vi "Afficheur - Copie.vi"() -> ()   [LabVIEW 2013]
uses:
  <vilib>/DAQmx/read.llb/DAQmx Read (Analog Wfm 1Chan NSamp).vi
  <vilib>/DAQmx/create/channels.llb/DAQmx Create Channel (AI-Voltage-Basic).vi
  <vilib>/DAQmx/configure/timing.llb/DAQmx Timing (Sample Clock).vi
  <vilib>/measure/matone.llb/Extract Single Tone Information 1 Chan.vi
  <vilib>/DAQmx/miscellaneous.llb/DAQmx Fill In Error Info.vi
  <vilib>/express/express analysis/Spectral/Block/exnSpectralBlock spectral measurements PSD poly.vi
  <vilib>/express/express analysis/Spectral/Block/exnSpectralBlock spectral measurements PSD WFM.vi
  <vilib>/express/express analysis/Spectral/XNode/ExpressSpectralMeasurementsBlockNode.xnode
  <vilib>/measure/NI_MAPro.lvlib
panel:
  out "indice fractionnaire ou x":dbl
  out "Y":dbl[](array[numeric])
  out "taille(s) 2":i32
  out "taille(s)":i32
  out "x*y":dbl
  out "Final Waveform":waveform(dbl)(graph)
  in  "TA":dbl
  out "signal 2":dbl[](graph)
  out "Valeur efficace":dbl
  out "?":cluster{"f0":dbl, "df":dbl, "magnitude":dbl[]}(graph)
  out "mean":dbl caption="moyenne" format="%0.2f"
  out "signal":waveform(dbl)(graph)
  out "Fréquence":dbl
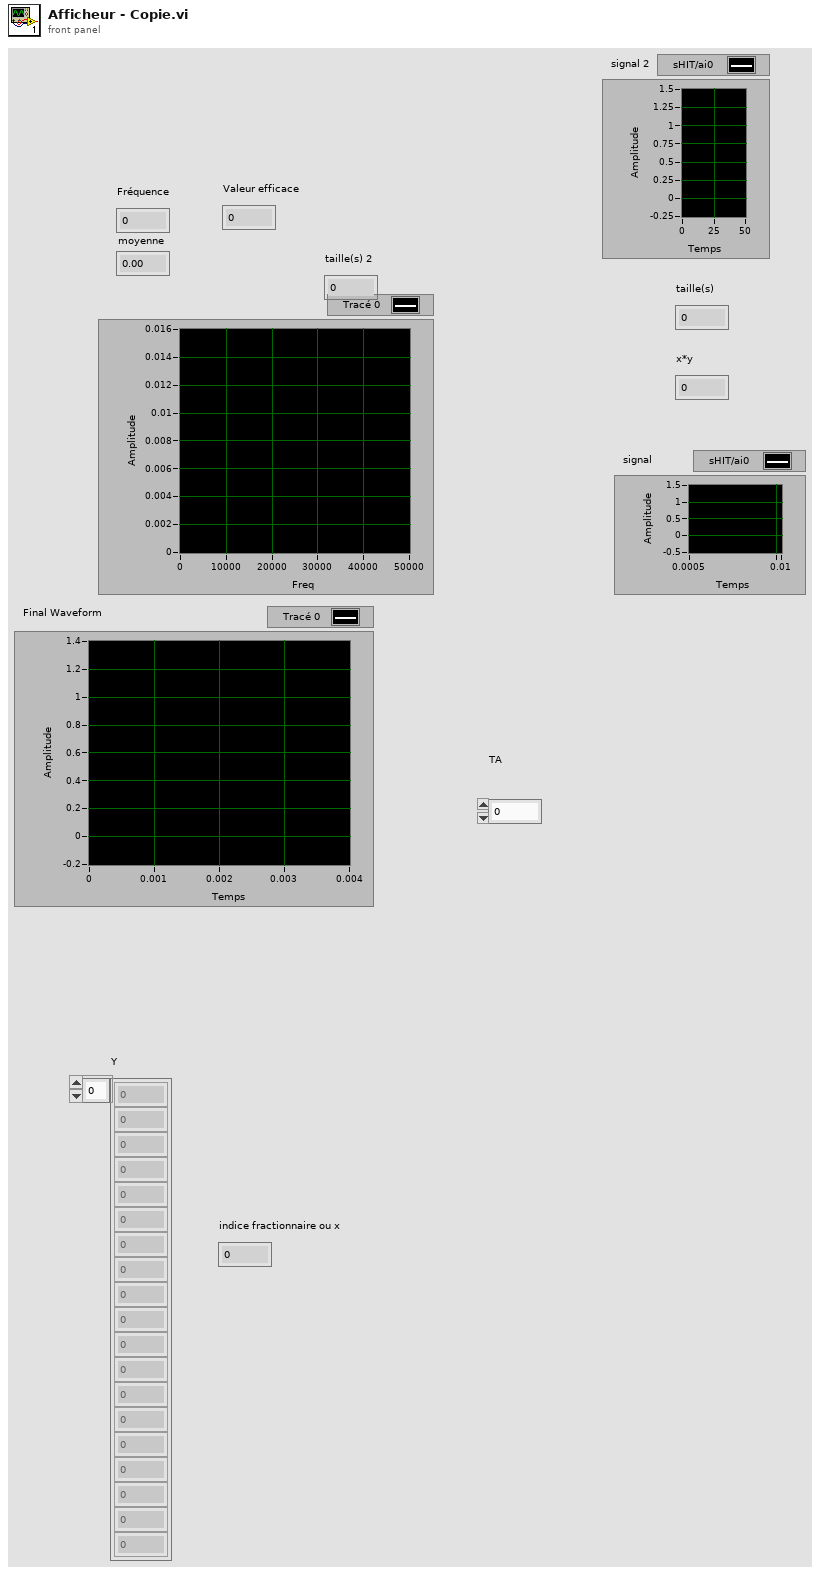
[diagram p1: front panel]
types:
  T1 = cluster{"averaging mode":u16, "weighting mode":u16, "number of averages":u32}
  T2 = cluster{"dB On (F)":bool, "unwrap phase (F)":bool, "convert to degree (F)":bool}
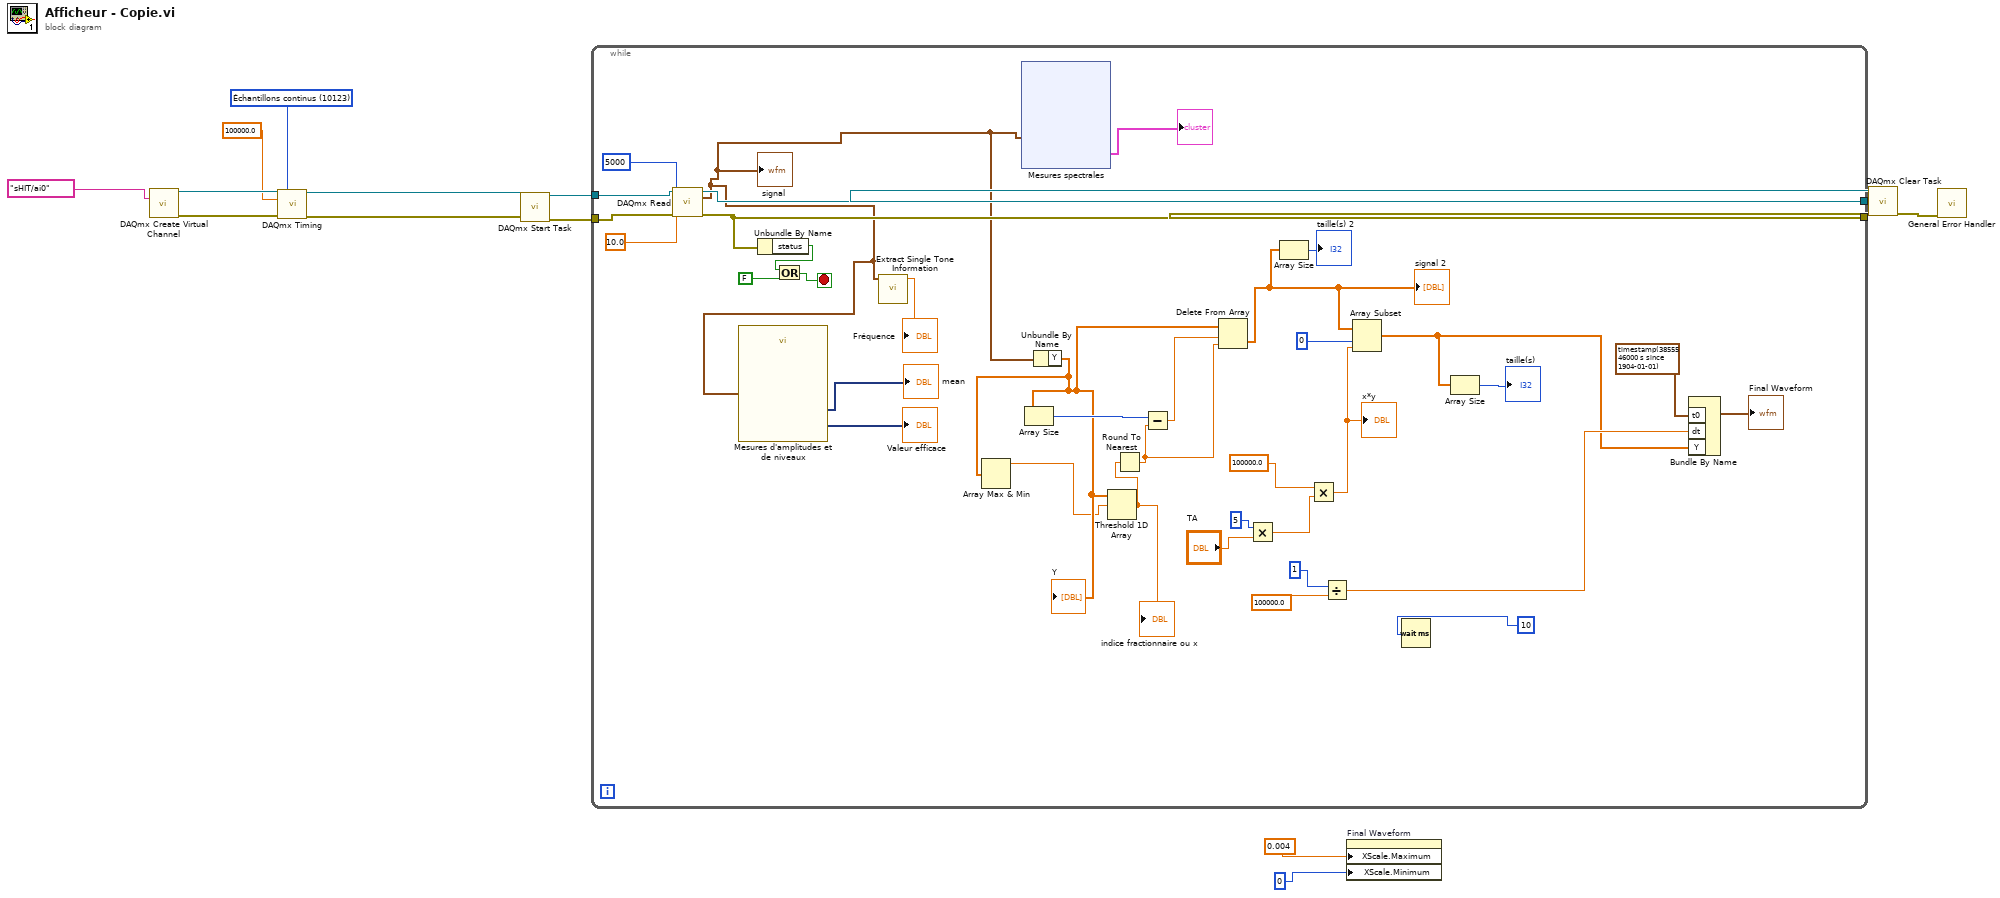
[diagram p0: block diagram]
diagram:
  w12 = 10123 items=["Échantillons finis"=10178, "Échantillons continus"=10123, "Point par point avec cadencement matériel"=12522] ("sample mode")
  n1 = call-poly <vilib>:"DAQmx Create Virtual Channel.vi"("physical channels"=tag "sHIT/ai0" ("Voie physique DAQmx")) -> ("task out"=w14:refnum<k21>, "error out"=w13:errorcluster)  [unwired: 13 in]
  n2 = call-poly <vilib>:"DAQmx Timing.vi"("task/channels in"=w14, "sample mode"=w12, "rate"=100000.0, "error in"=w13) -> ("task out"=w5:refnum<k21>, "error out"=w4:errorcluster)  [unwired: 10 in]
  n3 = call <vilib>:"DAQmx Start Task.vi"("task/channels in"=w5, "error in"=w4) -> ("task out"=w11:refnum<k21>, "error out"=w10:errorcluster)  [unwired: 12 in]
  n4 = while {
    tunnel: w11 -> [w50]
    tunnel: w10 -> [w49]
    tunnel: [w47] -> w9
    tunnel: [w43] -> w8
    stop <- w46 stop-if-true
    n5 = call-poly <vilib>:"DAQmx Read.vi"("task/channels in"=w50, "number of samples per channel"=5000, "timeout"=10.0, "error in"=w49) -> ("task out"=w47:refnum<k21>, "data"=w37:waveform(dbl), "error out"=w43:errorcluster)  [unwired: 9 in]
    "signal" <- w37
    n6 = call "Mesures d'amplitudes et de niveaux"("Signals"=w37) -> ("Mean (DC)"=→"mean":dynamicdata, "RMS"=→"Valeur efficace":dynamicdata)  [unwired: 12 in, 1 out]
    n7 = Unbundle By Name(w43) -> ("status"=w44:bool)
    n8 = Or(x=w44, y=FALSE) -> (x .or. y?=w46:bool)
    n9 = call-poly <vilib>:"Extract Single Tone Information.vi"("time signal in"=w37) -> ("detected frequency"=→"Fréquence":dbl)  [unwired: 5 in, 5 out]
    n10 = xnode "Mesures spectrales"("Signaux"=w37) -> ("DSP"=→"?":cluster{"f0":dbl, "df":dbl, "magnitude":dbl[]})  [unwired: 1 in, 1 out]
    n11 = Unbundle By Name(w37) -> ("Y"=w16:dbl[])
    "Y" <- w16
    n12 = Array Max & Min(array=w16) -> (max value=w15:dbl)  [unwired: 3 out]
    n13 = Array Size(array=w16) -> (size(s)=w36:i32)
    n14 = Threshold 1D Array(2:w15, 3:w16) -> (0:w21:dbl)  [unwired: 1 in]
    "indice fractionnaire ou x" <- w21
    n15 = Round To Nearest(number=w21) -> (nearest integer value=w20:dbl)
    n16 = Subtract(x=w36, y=w20) -> (x-y=w19:dbl)
    n17 = Delete From Array(array=w16, length=w19, index=w20) -> (deleted portion=w17:dbl[])  [unwired: 1 out]
    "signal 2" <- w17
    n18 = Multiply(x=5, y="TA") -> (x*y=w32:dbl)
    n19 = Array Size(array=w17) -> (size(s)=→"taille(s) 2":i32)
    n20 = Multiply(x=100000.0, y=w32) -> (x*y=w30:dbl)
    "x*y" <- w30
    n21 = Divide(x=1, y=100000.0) -> (x/y=w26:dbl)
    n22 = Array Subset(array=w17, index=0, length=w30) -> (w23:dbl[])
    n23 = Wait (ms)(milliseconds to wait=10) -> ()  [unwired: 1 out]
    n24 = Array Size(array=w23) -> (size(s)=→"taille(s)":i32)
    n25 = Bundle By Name("t0"=timestamp(3855546000 s since 1904-01-01), "dt"=w26, "Y"=w23) -> (→"Final Waveform":waveform(dbl))  [unwired: 1 in]
  }
  n26 = property on="Final Waveform" class="GraphWF (strict)"("XScale.Maximum"=0.004, "XScale.Minimum"=0) -> ()  [unwired: 2 in, 2 out]
  n27 = call <vilib>:"DAQmx Clear Task.vi"("task in"=w9, "error in"=w8) -> ("error out"=w7:errorcluster)  [unwired: 13 in]
  n28 = call <vilib>:"General Error Handler.vi"("error in (no error)"=w7) -> ()  [unwired: 10 in, 5 out]
